vi "Setpause.vi"(8 "error in (no error)":errorcluster, 10 "Pause":T1, 11 "PhotometricsCamIn":refnum<class "Photometrics_CH-250_Cam.lvclass">) -> (0 "error out":errorcluster, 3 "PhotometricsCamOut":refnum<class "Photometrics_CH-250_Cam.lvclass">)   [LabVIEW 2013, in "Photometrics_CH-250_Cam.lvclass"]
uses:
  Photometrics_CH-250_Cam.lvclass
  CameraSessionClass/CS250-CameraHardwareClass.lvclass
  shared/OnOffTypeDef.ctl
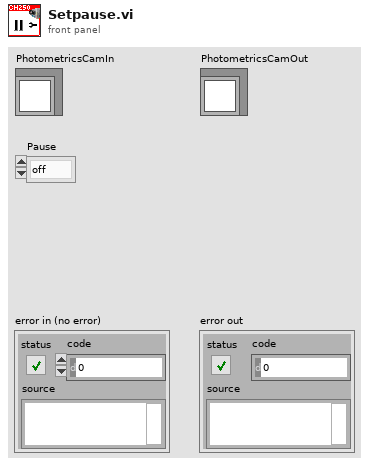
[diagram p1: front panel]
types:
  T1 = typedef "OnOffTypeDef.ctl" = enum16{"off", "on"}
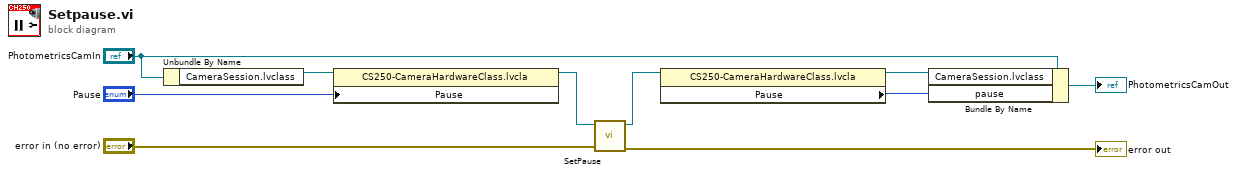
[diagram p0: block diagram]
diagram:
  n1 = Unbundle By Name("PhotometricsCamIn") -> ("CameraSession.lvclass"=w6:refnum<class "CS250-CameraHardwareClass.lvclass">)
  n2 = property class="CS250-CameraHardwareClass.lvcla"(reference=w6, "Pause"="Pause") -> (reference out=w5:refnum<class "CS250-CameraHardwareClass.lvclass">)  [unwired: 1 in, 1 out]
  n3 = call-dynamic "SetPause.vi"("error in (no error)"="error in (no error)", "CameraSession in"=w5) -> ("error out"=→"error out":errorcluster, "CameraSession out"=w3:refnum<class "CS250-CameraHardwareClass.lvclass">)  [unwired: 8 in]
  n4 = property class="CS250-CameraHardwareClass.lvcla"(reference=w3) -> (reference out=w2:refnum<class "CS250-CameraHardwareClass.lvclass">, "Pause"=w1:T1)  [unwired: 1 in, 1 out]
  n5 = Bundle By Name(cluster="PhotometricsCamIn", "CameraSession.lvclass"=w2, "pause"=w1) -> (→"PhotometricsCamOut":refnum<class "Photometrics_CH-250_Cam.lvclass">)
